vi "Copy State 1.vi"(7 "SourceCSM":refnum<class "CSM-Helper.lvclass">=refnum, 8 "error in (no error)":errorcluster, 9 "New(Empty to Use same Name)":string, 10 "Case":string="UI: Cursor Set", 11 "CSM-Helper.lvclass":refnum<class "CSM-Helper.lvclass">=refnum) -> (0 "error out":errorcluster, 3 "CSM-Helper out 2":refnum<class "CSM-Helper.lvclass">)   [LabVIEW 2020, in "CSM-Helper.lvclass"]
uses:
  CSM-Helper.lvclass
  <vilib>/Utility/miscctls.llb/LVPositionTypeDef.ctl
  CSM-Helper.lvclass/CSM-Helper.ctl
  Properties/Read Case Structure Ref.vi
  Get CaseFrame Reference By CaseName.vi
  Properties/Read Block Diagram Ref.vi
  Connect Internal Data Wire If not Connected.vi
  Connect StateQ Wire If not Connected.vi
  Set Error Tunnel Use Default If not Connected.vi
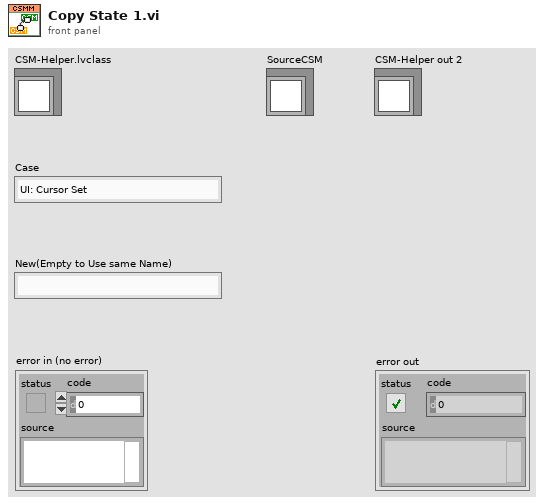
[diagram p1: front panel]
types:
  T1 = typedef "LVPositionTypeDef.ctl" = cluster{"Left":i32, "Top":i32}
  T2 = typedef "LVBoundsTypeDef.ctl" = cluster{"Width":u32, "Height":u32}
  T3 = cluster{"InternalData":refnum<vi>, "CSM Name":refnum<vi>, "Last Resp":refnum<vi>, "Remaining State":refnum<vi>, "Arguments":refnum<vi>, "Response Source":refnum<vi>, "Source CSM":refnum<vi>, "Selector":refnum<vi>, "Error":refnum<vi>}
  T4 = cluster{"InternalData":refnum<vi>, "Resp":refnum<vi>, "Remaining State":refnum<vi>, "Error":refnum<vi>}
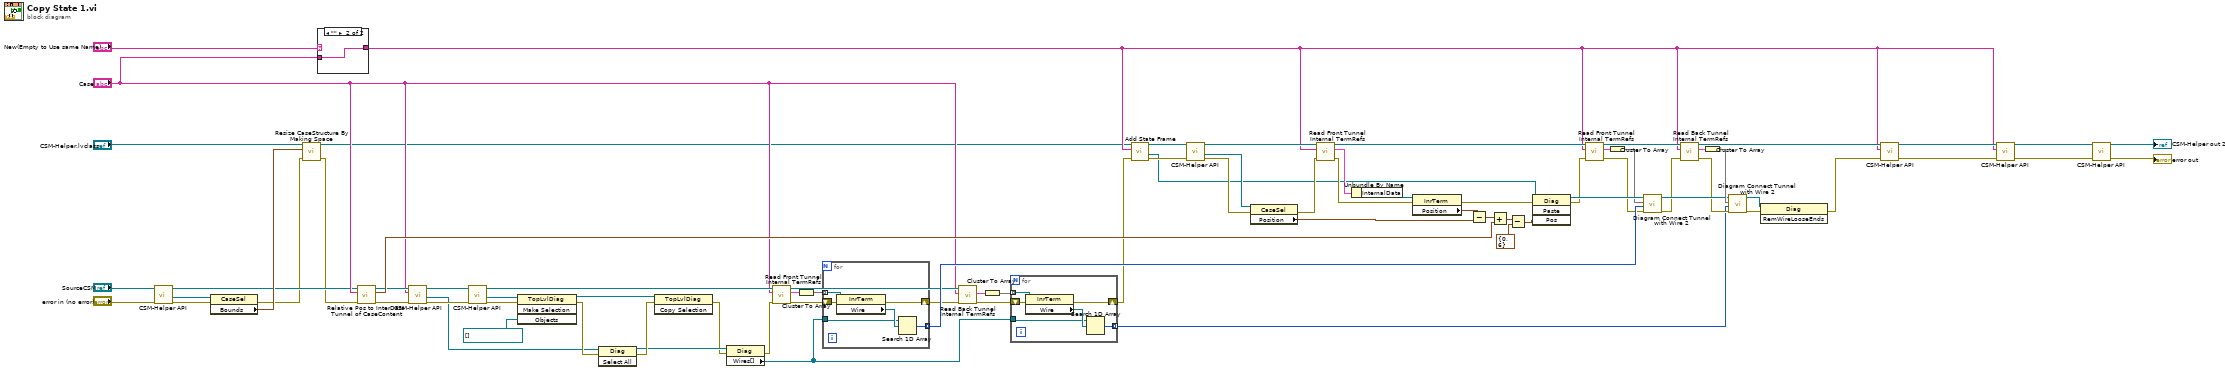
[diagram p0: block diagram]
diagram:
  n1 = call-poly "CSM-Helper API.vi"("error in (no error)"="error in (no error)", "CSM-Helper in"="SourceCSM") -> ("error out"=w12:errorcluster, "Case Structure"=w3:refnum<vi>, "CSM-Helper out"=w9:refnum<class "CSM-Helper.lvclass">)  [unwired: 7 in]
  n2 = property on="Property Node" class="CaseSel"(reference=w3, error in=w12) -> (error out=w8:errorcluster, "Bounds"=w14:T2)  [unwired: 1 out]
  n3 = call "Resize CaseStructure By Making Space.vi"("error in (no error)"=w8, "Bounds"=w14, "CSM-Helper in"="CSM-Helper.lvclass") -> ("error out"=w7:errorcluster, "CSM-Helper out"=w13:refnum<class "CSM-Helper.lvclass">)  [unwired: 5 in, 2 out]
  n4 = case shown="\"\"" "New(Empty to Use same Name)" {
    selector: "New(Empty to Use same Name)" -> [w81 _]
    tunnel: [w81 w82] -> w19
    tunnel: "Case" -> [_ w82]
    frame "False", Default {
    }
    frame "" {
    }
  }
  n5 = call "Relative Pos to InterData Tunnel of CaseContent.vi"("error in (no error)"=w7, "element"="Case", "CSM-Helper in"=w9) -> ("error out"=w25:errorcluster, "Position"=w57:T1, "CSM-Helper out"=w22:refnum<class "CSM-Helper.lvclass">)  [unwired: 6 in]
  n6 = call-poly "CSM-Helper API.vi"("error in (no error)"=w25, "CASE"="Case", "CSM-Helper in"=w22) -> ("error out"=w24:errorcluster, "Frame Refs"=w4:refnum<vi>, "CSM-Helper out"=w23:refnum<class "CSM-Helper.lvclass">)  [unwired: 6 in]
  n7 = call-poly "CSM-Helper API.vi"("error in (no error)"=w24, "CSM-Helper in"=w23) -> ("error out"=w17:errorcluster, "Diagram"=w5:refnum<vi>, "CSM-Helper out"=w68:refnum<class "CSM-Helper.lvclass">)  [unwired: 7 in]
  n8 = invoke on="Invoke Node" class="TopLvlDiag" method="Make Selection"(reference=w5, error in=w17, "Objects"=refnum<vi>[] []) -> (reference out=w16:refnum<vi>, error out=w18:errorcluster)  [unwired: 1 in, 2 out]
  n9 = invoke on="Invoke Node" class="Diag" method="Select All"(reference=w4, error in=w18) -> (reference out=w35:refnum<vi>, error out=w78:errorcluster)  [unwired: 1 in, 1 out]
  n10 = invoke on="Invoke Node" class="TopLvlDiag" method="Copy Selection"(reference=w16, error in=w78) -> (error out=w34:errorcluster)  [unwired: 1 in, 2 out]
  n11 = property on="Property Node" class="Diag"(reference=w35, error in=w34) -> (error out=w33:errorcluster, "Wires[]"=w28:refnum<vi>[])  [unwired: 1 out]
  n12 = call "Read Front Tunnel Internal TermRefs.vi"("error in (no error)"=w33, "case"="Case", "CSM-Helper in"=w68) -> ("error out"=w32:errorcluster, "Front Tunnels"=w74:T3, "CSM-Helper out"=w67:refnum<class "CSM-Helper.lvclass">)  [unwired: 6 in]
  n13 = Cluster To Array(cluster=w74) -> (array=w73:refnum<vi>[])
  n14 = for {
    tunnel: w28 -> [w87]
    tunnel: [w86] -> w75 mode=indexing
    tunnel: w73 -> [w85] mode=indexing
    shift-right: [w83] -> w31
    shift-left: w32 -> [w84]
    n15 = property class="InrTerm"(reference=w85, error in=w84) -> (error out=w83:errorcluster, "Wire"=w88:refnum<vi>)  [unwired: 1 out]
    n16 = Search 1D Array(1D array=w87, element=w88) -> (index of element=w86:i32)  [unwired: 1 in]
  }
  n17 = call "Read Back Tunnel Internal TermRefs.vi"("error in (no error)"=w31, "element"="Case", "CSM-Helper in"=w67) -> ("error out"=w29:errorcluster, "Front Tunnels"=w66:T4)  [unwired: 6 in, 1 out]
  n18 = Cluster To Array(cluster=w66) -> (array=w30:refnum<vi>[])
  n19 = for {
    tunnel: w28 -> [w93]
    tunnel: [w92] -> w26 mode=indexing
    tunnel: w30 -> [w91] mode=indexing
    shift-right: [w89] -> w27
    shift-left: w29 -> [w90]
    n20 = property class="InrTerm"(reference=w91, error in=w90) -> (error out=w89:errorcluster, "Wire"=w94:refnum<vi>)  [unwired: 1 out]
    n21 = Search 1D Array(1D array=w93, element=w94) -> (index of element=w92:i32)  [unwired: 1 in]
  }
  n22 = call "Add State Frame.vi"("error in (no error)"=w27, "element"=w19, "CSM-Helper in"=w13) -> ("error out"=w64:errorcluster, "Add Frame"=w1:refnum<vi>, "CSM-Helper out"=w79:refnum<class "CSM-Helper.lvclass">)  [unwired: 6 in]
  n23 = call-poly "CSM-Helper API.vi"("error in (no error)"=w64, "CSM-Helper in"=w79) -> ("error out"=w37:errorcluster, "Case Structure"=w2:refnum<vi>, "CSM-Helper out"=w65:refnum<class "CSM-Helper.lvclass">)  [unwired: 7 in]
  n24 = property on="Property Node" class="CaseSel"(reference=w2, error in=w37) -> (error out=w36:errorcluster, "Position"=w60:T1)  [unwired: 1 out]
  n25 = call "Read Front Tunnel Internal TermRefs.vi"("error in (no error)"=w36, "case"=w19, "CSM-Helper in"=w65) -> ("error out"=w76:errorcluster, "Front Tunnels"=w72:T3, "CSM-Helper out"=w70:refnum<class "CSM-Helper.lvclass">)  [unwired: 6 in]
  n26 = Unbundle By Name(w72) -> ("InternalData"=w80:refnum<vi>)
  n27 = property on="Property Node" class="InrTerm"(reference=w80, error in=w76) -> (error out=w77:errorcluster, "Position"=w61:T1)  [unwired: 1 out]
  n28 = Subtract(x=w61, y=w60) -> (x-y=w63:T1)
  n29 = Add(x=w63, y=w57) -> (x+y=w62:T1)
  n30 = Subtract(x=w62, y=T1 {"Left"=0, "Top"=6}) -> (x-y=w59:T1)
  n31 = invoke on="Invoke Node" class="Diag" method="Paste"(reference=w1, error in=w77, "Pos"=w59) -> (reference out=w71:refnum<vi>, error out=w69:errorcluster)  [unwired: 1 in, 2 out]
  n32 = call "Read Front Tunnel Internal TermRefs.vi"("error in (no error)"=w69, "case"=w19, "CSM-Helper in"=w70) -> ("error out"=w55:errorcluster, "Front Tunnels"=w54:T3, "CSM-Helper out"=w52:refnum<class "CSM-Helper.lvclass">)  [unwired: 6 in]
  n33 = Cluster To Array(cluster=w54) -> (array=w56:refnum<vi>[])
  n34 = call "Diagram Connect Tunnel with Wire 2.vi"("error in (no error)"=w55, "Wire Indexs"=w75, "Front Tunnels"=w56, "Diagram in"=w71) -> ("error out"=w45:errorcluster, "Diagram out"=w47:refnum<vi>)  [unwired: 5 in, 1 out]
  n35 = call "Read Back Tunnel Internal TermRefs.vi"("error in (no error)"=w45, "element"=w19, "CSM-Helper in"=w52) -> ("error out"=w44:errorcluster, "Front Tunnels"=w53:T4, "CSM-Helper out"=w51:refnum<class "CSM-Helper.lvclass">)  [unwired: 6 in]
  n36 = Cluster To Array(cluster=w53) -> (array=w48:refnum<vi>[])
  n37 = call "Diagram Connect Tunnel with Wire 2.vi"("error in (no error)"=w44, "Wire Indexs"=w26, "Front Tunnels"=w48, "Diagram in"=w47) -> ("error out"=w46:errorcluster, "Diagram out"=w40:refnum<vi>)  [unwired: 5 in, 1 out]
  n38 = invoke on="Invoke Node" class="Diag" method="RemWireLooseEnds"(reference=w40, error in=w46) -> (error out=w41:errorcluster)  [unwired: 1 in, 2 out]
  n39 = call-poly "CSM-Helper API.vi"("error in (no error)"=w41, "case"=w19, "CSM-Helper in"=w51) -> ("error out"=w50:errorcluster, "CSM-Helper out"=w49:refnum<class "CSM-Helper.lvclass">)  [unwired: 7 in]
  n40 = call-poly "CSM-Helper API.vi"("error in (no error)"=w50, "case"=w19, "CSM-Helper in"=w49) -> ("error out"=w42:errorcluster, "CSM-Helper out"=w43:refnum<class "CSM-Helper.lvclass">)  [unwired: 7 in]
  n41 = call-poly "CSM-Helper API.vi"("error in (no error)"=w42, "CSM-Helper in"=w43) -> ("error out"=→"error out":errorcluster, "CSM-Helper out"=→"CSM-Helper out 2":refnum<class "CSM-Helper.lvclass">)  [unwired: 8 in]
